vi "LCA Get Default Pos Unit.vi"(8 "error in (no error)":errorcluster caption="Fehler (Eingang, kein Fehler)", 11 "Axis Handle":i64) -> (0 "error out":errorcluster caption="Fehler (Ausgang)", 2 "Position Unit":i32, 3 "Prefix (milli, micro...)":i32)   [LabVIEW 2021, in "labbCAN_MotionControl_API.lvlib"]
doc: "LCA_Func long __stdcall LCA_GetDefaultPosUnit(dev_hdl hAxis,\n char* pPrefix,\n int* pPositionUnit);"
uses:
  labbCAN_MotionControl_API.lvlib
  labbCAN_MotionControl_API.dll
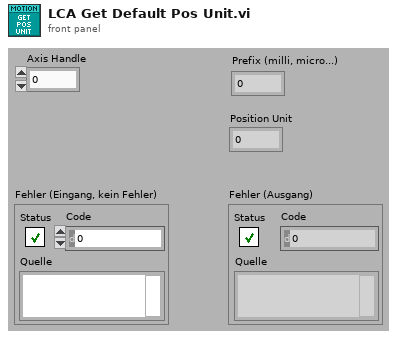
[diagram p1: front panel]
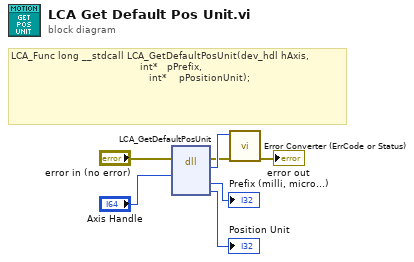
[diagram p0: block diagram]
diagram:
  # "LCA_Func long __stdcall LCA_GetDefaultPosUnit(dev_hdl hAxis,\n\t                                          int*   pPrefix,\n                                              int*    pPositionUnit);"
  n1 = dll-call lib="C:/Users/olaja/AppData/Local/CETONI_SDK/labbCAN_MotionControl_API.*" fn="LCA_GetDefaultPosUnit"(error in="error in (no error)", "hAxis"="Axis Handle") -> (error out=w3:errorcluster, "Rückgabetyp"=w4:i32, "pPrefix"=→"Prefix (milli, micro...)":i32, "pPositionUnit"=→"Position Unit":i32)  [unwired: 5 in, 1 out]
  n2 = call "Error Converter (ErrCode or Status).vi"("error in (no error)"=w3, "error code"=w4) -> ("error out"=→"error out":errorcluster)  [unwired: 9 in]
